vi "Proccess Lockin Channel.vi"(4 "Lock-in settings":T1={"Averaging period, s"=0.0, "Output Representation"=enum."Real/Imaginary", "Output value"=enum."RMS", "Phase delay, points"=0} {"Averaging period, s" format="%#_6p"}, 5 "Channel info":T2, 6 "Overwrite\nclock, Hz":dbl, 7 "Raw chunk size":i64, 8 "error in (no error)":errorcluster, 9 "Settings":string, 10 "group name":string, 11 "Data file path":path) -> (0 "error out":errorcluster, 1 "Settings out":string, 2 "Channel Length":u64, 3 "signal(s) out":waveform(dbl)[](array[waveform]))   [LabVIEW 2015]
uses:
  CH_name_pts_phase.ctl
  Syncronous Lockin Settings.ctl
  Utilities/Replace dt SGL.vi
  <vilib>/Waveform/WDTOps.llb/WDT Append Waveforms DBL.vi
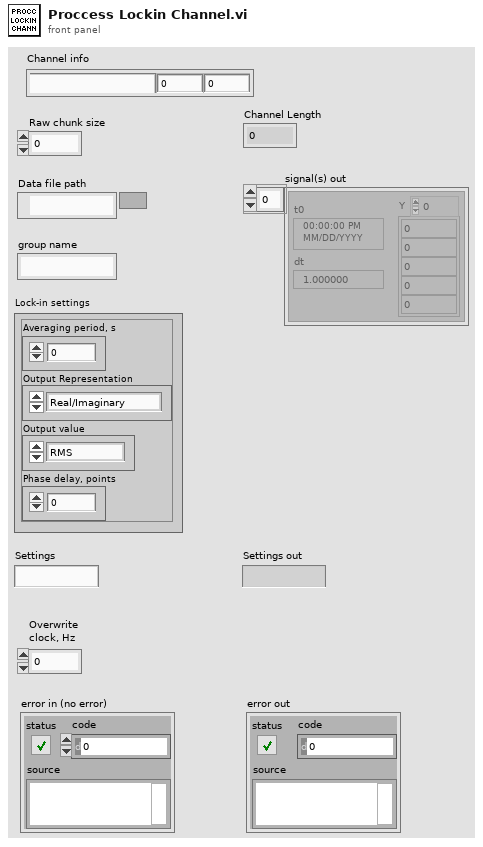
[diagram p1: front panel]
types:
  T1 = typedef "Syncronous Lockin Settings.ctl" = cluster{"Averaging period, s":dbl, "Output Representation":enum16{"Real/Imaginary", "Polar"}, "Output value":enum16{"Amplitude", "RMS", "Peak-to-Peak"}, "Phase delay, points":i32}
  T2 = typedef "CH_name_pts_phase.ctl" = cluster{"Channel":string, "pts per sine wave":i32, "Phase":dbl}
  T3 = enum16{"open", "open or create", "create or replace", "create", "open (read-only)"}
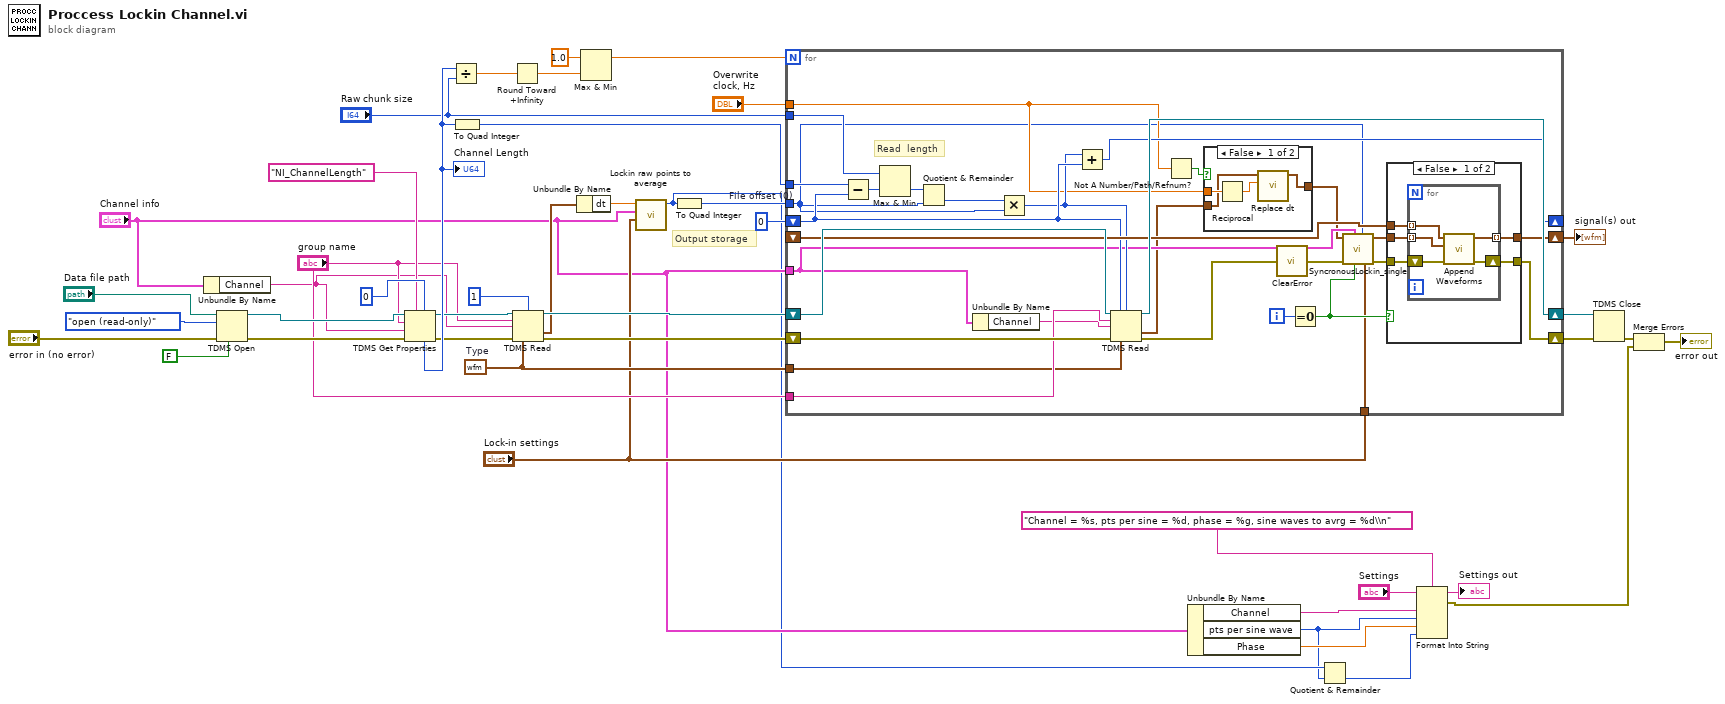
[diagram p0: block diagram]
diagram:
  w18 = waveform(sgl) {"t0"=timestamp(0 s since 1904-01-01), "dt"=1.0, "Y"=[]}  # Type
  w32 = i64 0  # File offset (0)
  # "Output storage"
  n1 = Unbundle By Name("Channel info") -> ("Channel"=w19:string)
  n2 = TDMS Open(6:FALSE ("disable buffering (T)"), 8:"error in (no error)", 10:T3."open (read-only)" ("TDMS open mode"), 11:"Data file path") -> (0:w28:errorcluster, 3:w29:refnum<k34>)  [unwired: 3 in]
  n3 = TDMS Get Properties(5:u64 0, 7:"NI_ChannelLength" ("property name"), 8:w28, 9:w19, 10:"group name", 11:w29) -> (0:w24:errorcluster, 3:w22:refnum<k34>, 4:w38:u64)  [unwired: 3 out]
  "Channel Length" <- w38
  n4 = Divide(x=w38, y="Raw chunk size") -> (x/y=w30:dbl)
  n5 = To Quad Integer(1:w38) -> (0:w39:i64)
  n6 = Round Toward +Infinity(x=w30) -> (ceil(x): smallest int >= x=w31:dbl)
  n7 = TDMS Read(0:w22, 2:i64 1 ("count (-1: all)"), 5:"group name", 7:w19, 11:w24, 12:w18) -> (4:w21:refnum<k34>, 10:w16:waveform(sgl), 15:w23:errorcluster)  [unwired: 2 in, 3 out]
  n8 = Unbundle By Name(w16) -> ("dt"=w15:dbl)
  n9 = Max & Min(x=1.0, y=w31) -> (max(x,y)=w36:dbl)  [unwired: 1 out]
  n10 = call "Lockin raw points to average.vi"("Lock-in settings"="Lock-in settings", "CH name                          points   phase"="Channel info", "dt"=w15) -> ("Lockin raw points to average"=w2:i32)  [unwired: 8 in]
  n11 = To Quad Integer(1:w2) -> (0:w40:i64)
  n12 = for {
    N: w36 -> [_]
    shift-right: [w61] -> w13
    shift-left: w23 -> [w74]
    shift-right: [w71] -> w34
    shift-left: w21 -> [w73]
    tunnel: "group name" -> [w72]
    tunnel: "Channel info" -> [w50]
    shift-right: [w70] -> _
    shift-left: w32 -> [w60]
    tunnel: "Raw chunk size" -> [w54]
    tunnel: w18 -> [w69]
    shift-right: [w66] -> w43
    shift-left: _ -> [w65]
    tunnel: w40 -> [w46]
    tunnel: w39 -> [w55]
    tunnel: "Overwrite\nclock, Hz" -> [w53]
    tunnel: "Lock-in settings" -> [w45]
    i -> [w67]
    # "Read  length"
    n13 = Subtract(x=w55, y=w60) -> (x-y=w59:i64)
    n14 = Max & Min(x=w54, y=w59) -> (min(x,y)=w58:i64)  [unwired: 1 out]
    n15 = Quotient & Remainder(x=w58, y=w46) -> (floor(x/y)=w57:i64)  [unwired: 1 out]
    n16 = Unbundle By Name(w50) -> ("Channel"=w51:string)
    n17 = Multiply(x=w57, y=w46) -> (x*y=w56:i64)
    n18 = Add(x=w56, y=w60) -> (x+y=w70:i64)
    n19 = TDMS Read(0:w73, 1:w60, 2:w56, 5:w72, 7:w51, 11:w74, 12:w69) -> (4:w71:refnum<k34>, 10:w48:waveform(sgl), 15:w52:errorcluster)  [unwired: 1 in, 3 out]
    n20 = Not A Number/Path/Refnum?(number/path/refnum=w53) -> (NaN/Path/Refnum?=w49:bool)
    n21 = case shown="False" w49 {
      tunnel: w48 -> [w76 w79]
      tunnel: [w78 w79] -> w47
      tunnel: w53 -> [w77 _]
      frame False {
        n22 = Reciprocal(x=w77) -> (1/x=w75:dbl)
        n23 = call-poly "Replace dt.vi"("dt"=w75, "Waveform in"=w76) -> ("Waveform out"=w78:waveform(sgl))  [unwired: 9 in]
      }
      frame True {
      }
    }
    n24 = call <vilib>:"ClearError.vi"("error in (no error)"=w52) -> ("error out"=w68:errorcluster)
    n25 = Equal To 0?(x=w67) -> (x = 0?=w64:bool)
    n26 = call "SyncronousLockin_single.vi"("Lock-in settings"=w45, "Raw points to average"=w46, "First chunk?"=w64, "CH name                          points   phase"=w50, "error in (no error)"=w68, "Data"=w47) -> ("error out"=w63:errorcluster, "signal(s) out"=w62:waveform(dbl)[])  [unwired: 4 in]
    n27 = case shown="False" w64 {
      tunnel: [w84 w91] -> w66
      tunnel: w65 -> [w82 _]
      tunnel: w63 -> [w83 w90]
      tunnel: w62 -> [w81 w91]
      tunnel: [w80 w90] -> w61
      frame False {
        n28 = for {
          tunnel: [w89] -> w84 mode=indexing
          tunnel: w82 -> [w88] mode=indexing
          shift-right: [w86] -> w80
          shift-left: w83 -> [w87]
          tunnel: w81 -> [w85] mode=indexing
          n29 = call-poly <vilib>:"Append Waveforms.vi"("error in (no error)"=w87, "waveform B"=w85, "waveform A"=w88) -> ("error out"=w86:errorcluster, "waveform out"=w89:waveform(dbl))  [unwired: 7 out]
        }
      }
      frame True {
      }
    }
  }
  "signal(s) out" <- w43
  n30 = Unbundle By Name("Channel info") -> ("Channel"=w9:string, "pts per sine wave"=w1:i32, "Phase"=w8:dbl)
  n31 = Quotient & Remainder(x=w2, y=w1) -> (floor(x/y)=w3:i32)  [unwired: 1 out]
  n32 = Format Into String(format string="Channel = %s, pts per sine = %d, phase = %g, sine waves to avrg = %d\\n", initial string="Settings", w9, w1, w8, w3) -> (resulting string=→"Settings out":string, error out=w4:errorcluster)  [unwired: 1 in]
  n33 = TDMS Close(8:w13, 11:w34) -> (0:w12:errorcluster)  [unwired: 1 out]
  n34 = Merge Errors(w12, w4) -> (→"error out":errorcluster)
